vi "delete_data.vi"(10 "table":string, 11 "condition":string) -> (0 "connection reference out":T1, 1 "Application Directory":path, 2 "connection information":path, 3 "error out":errorcluster)   [LabVIEW 2014]
doc: "This Block is used to delete certain data from Database Table based on the Condition.\n\nit takes 2 arguments representing table name and condition."
uses:
  <vilib>/addons/database/Connection.llb/Conn ObjectReference.ctl
  <vilib>/addons/database/Connection.llb/DB Tools Open Connec (Path).vi
  <vilib>/addons/database/NI_Database_API.lvlib
panel:
  # "This Block is used to delete certain data from Database Table"
  # "Inputs"
  # "Outputs"
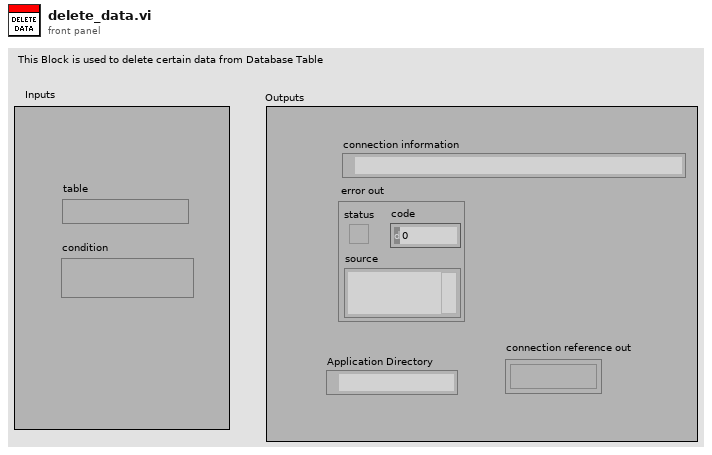
[diagram p1: front panel]
types:
  T1 = typedef "NI_Database_API.lvlib/Conn ObjectReference.ctl" = refnum<k1>
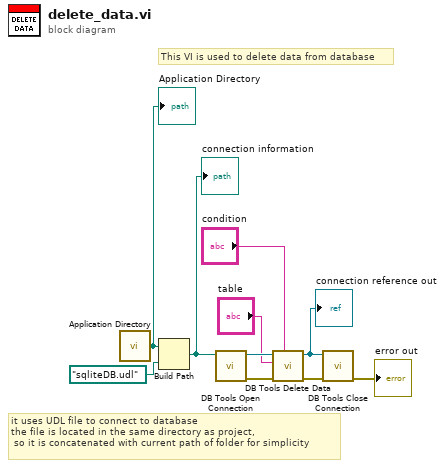
[diagram p0: block diagram]
diagram:
  # "it uses UDL file to connect to database\nthe file is located in the same directory as project,\n so it is concatenated with current path of folder for simplicity"
  # "This VI is used to delete data from database"
  n1 = call <vilib>:"Application Directory.vi"() -> ("Application Directory"=w8:path)
  "Application Directory" <- w8
  n2 = Build Path(base path=w8, name or relative path=path "sqliteDB.udl" ("connection information")) -> (appended path=w7:path)
  "connection information" <- w7
  n3 = call-poly <vilib>:"DB Tools Open Connection.vi"("connection information"=w7) -> ("error out"=w9:errorcluster, "connection reference"=w10:T1)  [unwired: 7 in]
  n4 = call <vilib>:"DB Tools Delete Data.vi"("condition"="condition", "error in (no error)"=w9, "table"="table", "connection reference"=w10) -> ("error out"=w3:errorcluster, "connection reference out"=w4:T1)  [unwired: 6 in]
  "connection reference out" <- w4
  n5 = call <vilib>:"DB Tools Close Connection.vi"("error in (no error)"=w3, "connection reference"=w4) -> ("error out"=→"error out":errorcluster)  [unwired: 5 in]
